vi "Convert Modular CALs to Full System CAL.vi"() -> ()   [LabVIEW 2011]
uses:
  WebEngine/LIB/MODULES/Module_Types.ctl
  WebEngine/LIB/MODULES/ModuleDef.ctl
  WebEngine/LIB/MODULES/RF Module/RF Module Parameters.ctl
  WebEngine/LIB/MODULES/PA Module/PA Module Parameters.ctl
  WebEngine/LIB/MODULES/FE Module/FE Module Parameters.ctl
  WebEngine/LIB/MODULES/SW Module/SW Module Parameters.ctl
  WebEngine/LIB/MODULES/TestSetModules.ctl
panel:
  out "error out":errorcluster
  in  "FEModule CAL File":path
  in  "PAModule CAL File":path
  in  "RFModule CAL File":path
  in  "error in (no error)":errorcluster
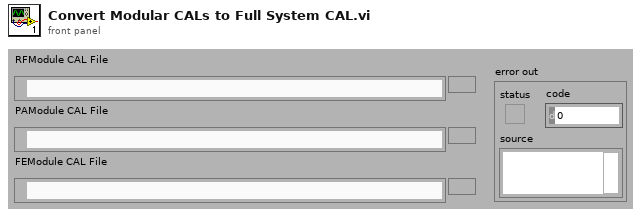
[diagram p1: front panel]
types:
  T1 = typedef "TestSetModules.ctl" = cluster{"RFModule":T2, "PAModule":T5, "FEModule":T6, "SW Modules":T7[]}
  T2 = typedef "RF Module Parameters.ctl" = cluster{"ID":u16, "Model":string, "Device":T3, "Parameters":cluster{"SYBandsCount":i32, "SYBands":cluster{"Fstart":dbl, "Fstop":dbl, "Fstep":dbl}[]}}
  T3 = typedef "ModuleDef.ctl" = cluster{"DevName":string, "DevDetails":string, "DevID":u32, "HW Present":bool, "Module ID":u16, "ModuleCAL":path, "Module Type":T4, "Valid Cal?":bool, "UID":string}
  T4 = typedef "Module_Types.ctl" = enum16{"Unknown", "RF Module", "PA Module", "TR Module", "FE Module", "SW Module"}
  T5 = typedef "PA Module Parameters.ctl" = cluster{"ID":u16, "Model":string, "Device":T3, "Parameters":cluster{"Band":cluster{"Fstart":dbl, "Fstop":dbl}, "Pstep":dbl, "MinAtten":dbl, "MinAttenOptH":dbl}, "Options":cluster{"H":bool}}
  T6 = typedef "FE Module Parameters.ctl" = cluster{"ID":u16, "Model":string, "Device":T3, "Parameters":cluster{"Tx1":cluster{"Fstart":dbl, "Fstop":dbl}, "Tx2":cluster{"Fstart":dbl, "Fstop":dbl}, "Rx":cluster{"Fstart":dbl, "Fstop":dbl}, "LowSide?":bool}, "Options":cluster{"B":bool, "F":bool, "D":bool}}
  T7 = typedef "SW Module Parameters.ctl" = cluster{"ID":u16, "Model":string, "Device":T3, "Parameters":cluster{"COM Dev":string, "TX Devs":string[], "RX Devs":string[]}}
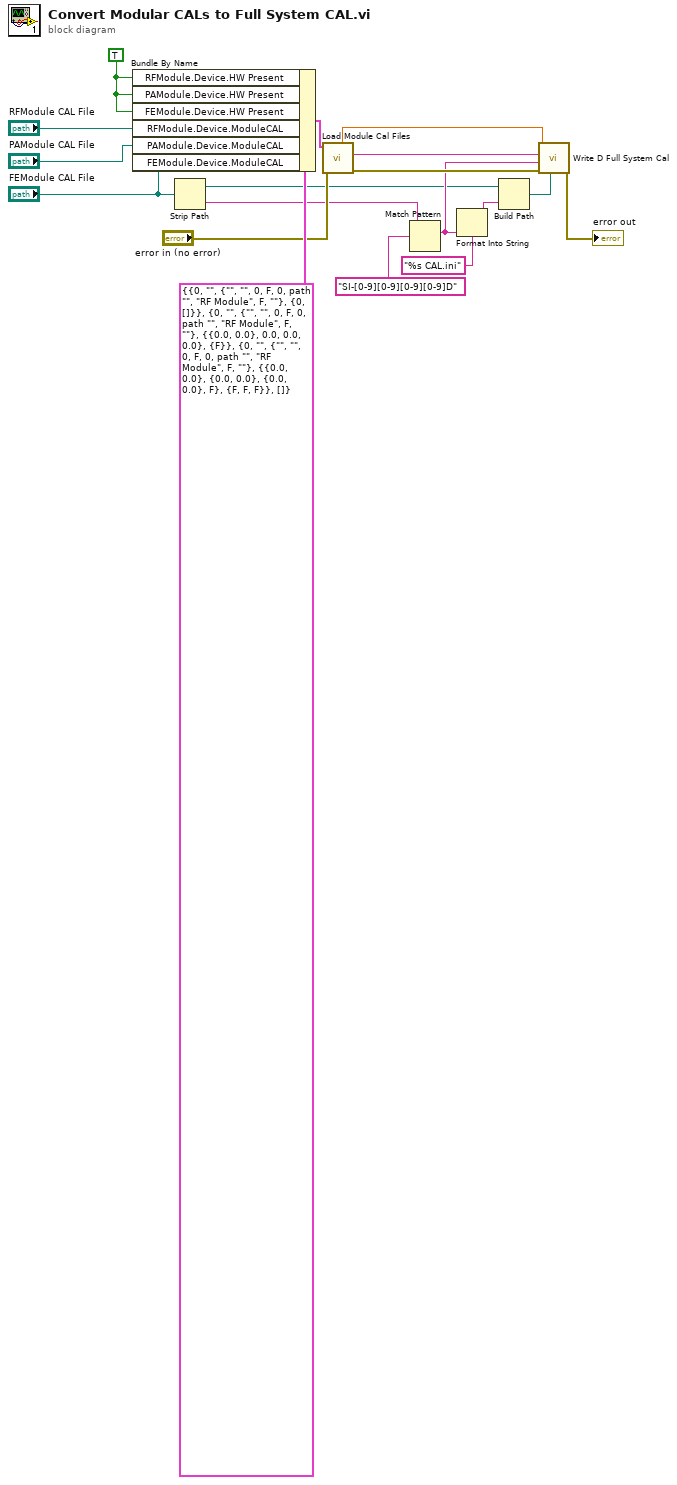
[diagram p0: block diagram]
diagram:
  w1 = TRUE
  n1 = Bundle By Name(cluster=T1 {"RFModule"={"ID"=0, "Model"="", "Device"={"DevName"="", "DevDetails"="", "DevID"=0, "HW Present"=FALSE, "Module ID"=0, "ModuleCAL"=path "", "Module Type"=enum."RF Module", "Valid Cal?"=FALSE, "UID"=""}, "Parameters"={"SYBandsCount"=0, "SYBands"=[]}}, "PAModule"={"ID"=0, "Model"="", "Device"={"DevName"="", "DevDetails"="", "DevID"=0, "HW Present"=FALSE, "Module ID"=0, "ModuleCAL"=path "", "Module Type"=enum."RF Module", "Valid Cal?"=FALSE, "UID"=""}, "Parameters"={"Band"={"Fstart"=0.0, "Fstop"=0.0}, "Pstep"=0.0, "MinAtten"=0.0, "MinAttenOptH"=0.0}, "Options"={"H"=FALSE}}, "FEModule"={"ID"=0, "Model"="", "Device"={"DevName"="", "DevDetails"="", "DevID"=0, "HW Present"=FALSE, "Module ID"=0, "ModuleCAL"=path "", "Module Type"=enum."RF Module", "Valid Cal?"=FALSE, "UID"=""}, "Parameters"={"Tx1"={"Fstart"=0.0, "Fstop"=0.0}, "Tx2"={"Fstart"=0.0, "Fstop"=0.0}, "Rx"={"Fstart"=0.0, "Fstop"=0.0}, "LowSide?"=FALSE}, "Options"={"B"=FALSE, "F"=FALSE, "D"=FALSE}}, "SW Modules"=[]} ("Modules"), "RFModule.Device.HW Present"=w1, "PAModule.Device.HW Present"=w1, "FEModule.Device.HW Present"=w1, "RFModule.Device.ModuleCAL"="RFModule CAL File", "PAModule.Device.ModuleCAL"="PAModule CAL File", "FEModule.Device.ModuleCAL"="FEModule CAL File") -> (w17:T1)
  n2 = Strip Path(path="FEModule CAL File") -> (stripped path=w6:path, name=w10:string)
  n3 = call "Load Module Cal Files.vi"("error in (no error)"="error in (no error)", 11:w17) -> ("error out"=w14:errorcluster, "Cal Serial Number"=w12:string, "Cal DateDBL"=w13:dbl)  [unwired: 6 in, 1 out]
  n4 = Match Pattern(string=w10, regular expression="SI-[0-9][0-9][0-9][0-9]D") -> (match substring=w8:string)  [unwired: 1 in, 3 out]
  n5 = Format Into String(format string="%s CAL.ini", w8) -> (resulting string=w7:string)  [unwired: 2 in, 1 out]
  n6 = Build Path(base path=w6, name or relative path=w7) -> (appended path=w5:path)
  n7 = call "Write D Full System Cal.vi"("Cal File Path"=w5, "error in (no error)"=w14, "Model"=w8, "Cal Serial Number"=w12, "Cal DateDBL"=w13) -> ("error out"=→"error out":errorcluster)  [unwired: 6 in]
